vi "monitor_odczyt 2.vi"(10 "output cluster":T2 {"Cluster"."array of cans"."type" items=["CAN Data", "CAN Remote"]; "Cluster"."array of cans"."identifier" format="%.0x"}) -> (0 "ramki jazdy out":T1[](array[typedef]) {"type" items=["CAN Data", "CAN Remote"]; "identifier" format="%.0x"}, 1 "Delay":dbl, 3 "Przestarza³a data":bool caption="Time has Elapsed")   [LabVIEW 2015]
uses:
  <vilib>/Utility/Variable/NI_VariableUtilities.lvlib
  <vilib>/RioEmbeddedCAN/RioEmbeddedCAN.llb/CANFrameControl.ctl
panel:
  in  "TIME_SBRIO 2":timestamp format="%<%H:%M:%S%1u>T"
  out "x+y":timestamp
  out "TIME_DATA":timestamp format="%<%H:%M:%S%1u>T"
  out "TIME_SBRIO":timestamp format="%<%H:%M:%S%1u>T"
  in  "ramki jazdy zerowanie":T1[](array[typedef])=[{"identifier"=1, "extended?"=FALSE, "type"=0, "payload"=[1, 127, 255, 127, 255, 127, 255, 0]}, {"identifier"=2, "extended?"=FALSE, "type"=0, "payload"=[1, 127, 255, 127, 255, 127, 255, 0]}] {"type" items=["CAN Data", "CAN Remote"]; "identifier" format="%.0x"}
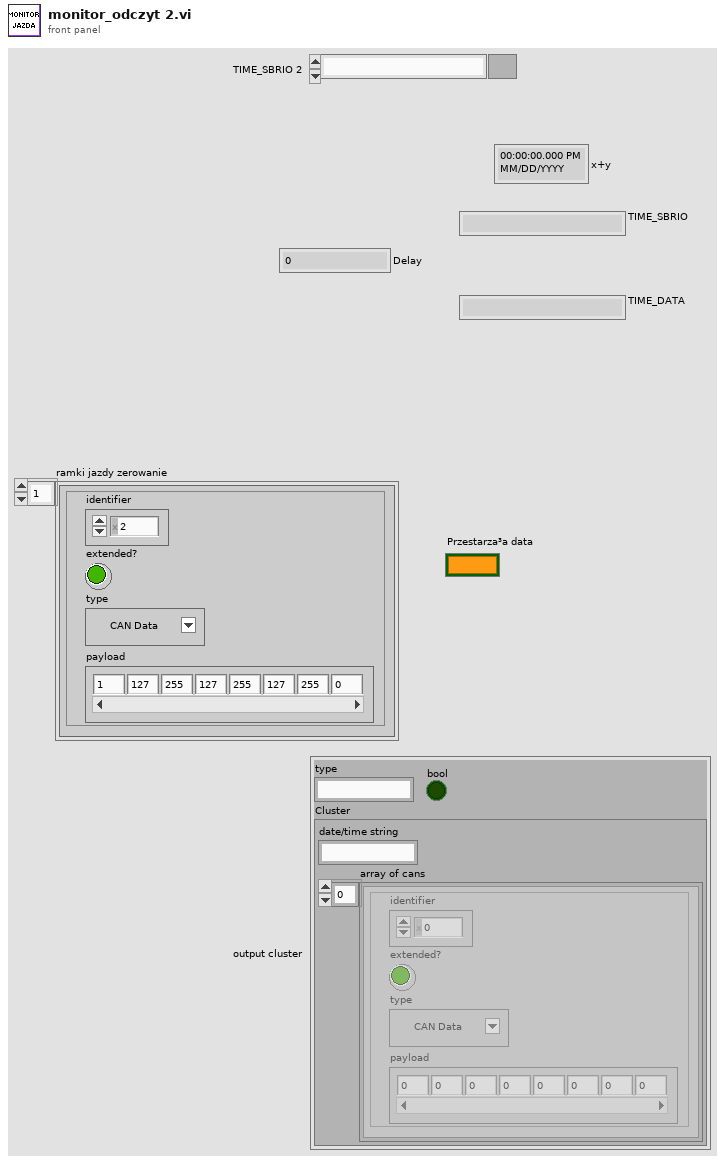
[diagram p1: front panel]
types:
  T1 = typedef "CANFrameControl.ctl" = cluster{"identifier":u32, "extended?":bool, "type":u8, "payload":u8[]}
  T2 = cluster{"type":string, "Cluster":cluster{"date/time string":string, "array of cans":T1[]}, "bool":bool}
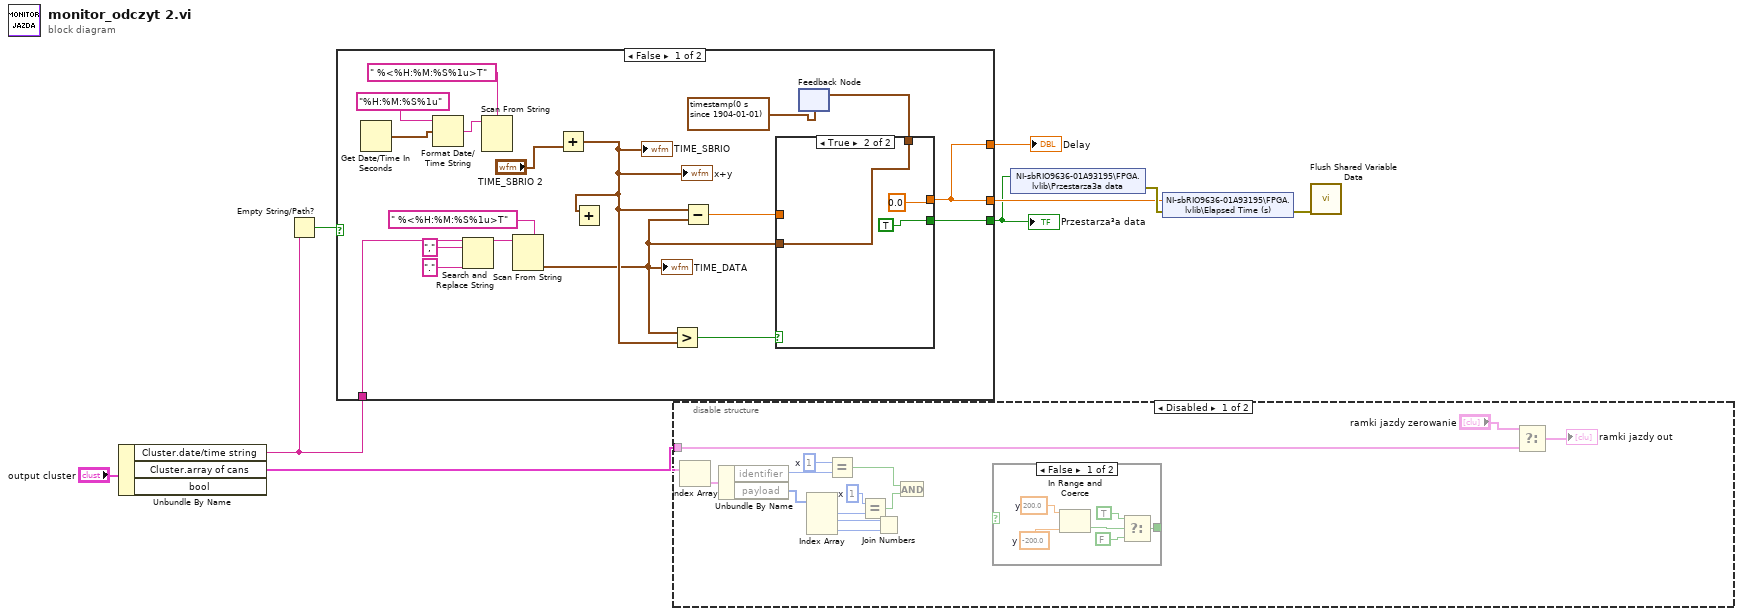
[diagram p0: block diagram]
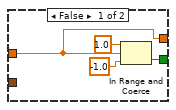
[diagram p2: hidden frame]
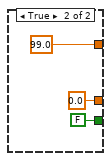
[diagram p3: hidden frame]
diagram:
  n1 = Unbundle By Name("output cluster") -> ("Cluster.date/time string"=w4:string, "Cluster.array of cans"=w7:T1[])  [unwired: 1 out]
  n2 = Empty String/Path?(string/path=w4) -> (empty?=w3:bool)
  n3 = case shown="False" w3 {
    tunnel: [w20 0.0] -> w6
    tunnel: [w19 FALSE] -> w5
    tunnel: w4 -> [w25 _]
    tunnel: [w20 99.0] -> w2
    frame False {
      n4 = Get Date/Time In Seconds() -> (seconds since 1Jan1904=w13:timestamp)
      n5 = Format Date/Time String(time format string (%c)="%H:%M:%S%1u", seconds (now)=w13) -> (date/time string=w23:string)  [unwired: 1 in]
      n6 = Search and Replace String(input string=w25, search string=",", replace string="." ("replace string (\"\")")) -> (result string=w26:string)  [unwired: 5 in, 3 out]
      n7 = Scan From String(format string=" %<%H:%M:%S%1u>T" ("time format string (%c)"), input string=w23) -> ()  [unwired: 4 in, 3 out]
      n8 = Scan From String(format string=" %<%H:%M:%S%1u>T" ("time format string (%c)"), input string=w26) -> (output 1=w10:timestamp)  [unwired: 3 in, 3 out]
      "TIME_DATA" <- w10
      n9 = Add(y="TIME_SBRIO 2") -> (x+y=w11:timestamp)  [unwired: 1 in]
      "TIME_SBRIO" <- w11
      "x+y" <- w11
      n10 = Add(x=w11) -> ()  [unwired: 1 in, 1 out]
      n11 = Greater?(x=w10, y=w11) -> (0:w21:bool)
      n12 = Subtract(x=w11, y=w10) -> (x-y=w22:dbl)
      n13 = case shown="True" w21 {
        tunnel: [w30 TRUE] -> w19
        tunnel: w22 -> [w29 _]
        tunnel: [w29 0.0] -> w20
        tunnel: [_ w33] -> w16
        tunnel: w10 -> [_ w33]
        frame False {
          n14 = In Range and Coerce(upper limit=1.0, x=w29, lower limit=-1.0 ("upper limit")) -> (In Range?=w30:bool)  [unwired: 1 out]
        }
        frame True {
        }
      }
      n15 = feedback-in #1(w16) -> ()
      n16 = feedback #1(timestamp(0 s since 1904-01-01) ("output 1")) -> (w14:timestamp)
    }
    frame True {
    }
  }
  "Przestarza³a data" <- w5
  "Delay" <- w2
  n17 = disable-structure shown="Disabled" {
    disable-tunnel: w7 -> [w40 _]
    frame Disabled {
      w47 = u8 1  # x
      w49 = u32 1  # x
      n18 = Index Array(array=w40) -> (element=w51:T1)  [unwired: 1 in]
      n19 = Unbundle By Name(w51) -> ("identifier"=w50:u32, "payload"=w39:u8[])
      n20 = Index Array(array=w39) -> (element #1=w48:u8, element #2=w46:u8, element #3=w45:u8)  [unwired: 3 in]
      n21 = Equal?(x=w49, y=w50) -> (x = y?=w44:bool)
      n22 = Equal?(x=w47, y=w48) -> (x = y?=w43:bool)
      n23 = Join Numbers(hi=w46, lo=w45) -> ()  [unwired: 1 out]
      n24 = And(x=w44, y=w43) -> ()  [unwired: 1 out]
      n25 = case shown="False" {
        selector: _ -> [_ _]
        tunnel: [w55 _] -> _
        frame False {
          w56 = 200.0  # y
          w57 = -200.0  # y
          n26 = In Range and Coerce(upper limit=w56, lower limit=w57) -> (In Range?=w52:bool)  [unwired: 1 in, 1 out]
          n27 = Select(t=TRUE, s=w52, f=FALSE) -> (s? t:f=w55:bool)
        }
        frame True {
        }
      }
      n28 = Select(t="ramki jazdy zerowanie", f=w40) -> (s? t:f=→"ramki jazdy out":T1[])  [unwired: 1 in]
    }
    frame Enabled {
    }
  }
  n29 = shared-variable "NI-sbRIO9636-01A93195\\FPGA.lvlib\\Przestarza3a data"(w5) -> (error out=w9:errorcluster)  [unwired: 1 in]
  n30 = shared-variable "NI-sbRIO9636-01A93195\\FPGA.lvlib\\Elapsed Time (s)"(w6, error in=w9) -> (error out=w8:errorcluster)
  n31 = call <vilib>:"Flush Shared Variable Data.vi"("error in (no error)"=w8) -> ()  [unwired: 10 in, 1 out]
